vi "creator_map_write.vi"(8 "error in":errorcluster, 10 "creator map":map{string, T1}(c390), 11 "file path":path) -> (0 "error out":errorcluster)   [LabVIEW 2024, in "MemoryManager.lvclass"]
uses:
  MemoryManager.lvclass
  MemoryManager.lvclass/MemoryManager.ctl
  creator_map_value--cluster.ctl
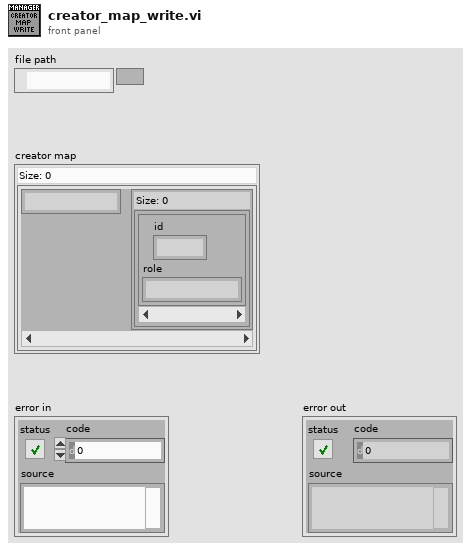
[diagram p1: front panel]
types:
  T1 = typedef "MemoryManager.lvclass/creator_map_value--cluster.ctl" = set{cluster{"id":i32, "role":string}}
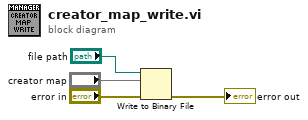
[diagram p0: block diagram]
diagram:
  n1 = Write to Binary File(file (use dialog)="file path", data="creator map", error in="error in") -> (error out=→"error out":errorcluster)  [unwired: 3 in, 2 out]
